vi "Table Buffer - Dequeue.vi"(8 "error in (no error)":errorcluster) -> (0 "error out":errorcluster, 3 "Data":string[][](array[string]))   [LabVIEW 2025, in "I2C Bus Monitor UI.lvlib"]
uses:
  I2C Bus Monitor UI.lvlib
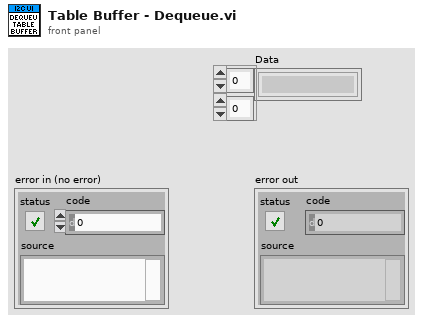
[diagram p1: front panel]
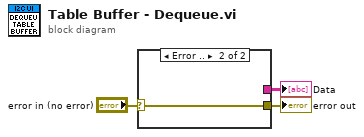
[diagram p0: block diagram]
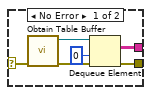
[diagram p2: hidden frame]
diagram:
  n1 = case shown="Error .." "error in (no error)" {
    selector: "error in (no error)" -> [w9 w10]
    tunnel: [w8 w10] -> w2
    tunnel: [w7 _] -> w1
    frame No Error {
      n2 = call "Obtain Table Buffer.vi"("error in (no error)"=w9) -> ("error out"=w5:errorcluster, "Table Queue"=w4:refnum<queue>)  [unwired: 9 in]
      n3 = Dequeue Element(queue=w4, timeout in ms (-1)=0, error in (no error)=w5) -> (element=w7:string[][], error out=w8:errorcluster)  [unwired: 2 out]
    }
    frame Error {
    }
  }
  "error out" <- w2
  "Data" <- w1
